vi "Start Asynchronous Error Msg.vi"(8 "error in (no error)":errorcluster, 10 "throw msg?":bool, 11 "eMsg":string) -> (0 "error out":errorcluster)   [LabVIEW 2012]
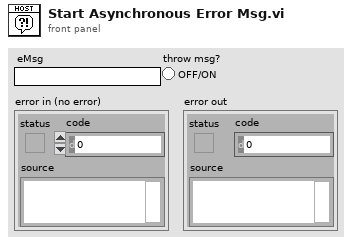
[diagram p1: front panel]
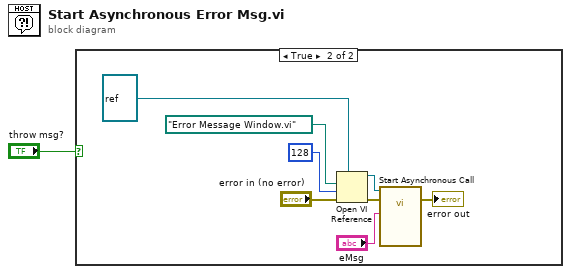
[diagram p0: block diagram]
diagram:
  n1 = case shown="True" "throw msg?" {
    frame False {
    }
    frame True {
      n2 = Open VI Reference(type specifier VI Refnum (for type only)=refnum<vi> refnum, vi path=path "Error Message Window.vi", options=128, error in (no error)="error in (no error)") -> (vi reference=w7:refnum<vi>, error out=w6:errorcluster)  [unwired: 2 in]
      n3 = call-by-ref "Start Asynchronous Call"(reference=w7, error in=w6, "eMsg"="eMsg") -> (error out=→"error out":errorcluster)  [unwired: 11 in, 1 out]
    }
  }
